vi "Template UIP Path.vi"() -> (3 "Template UIP Path":path)   [LabVIEW 2020, in "UIM.lvlib" / "UIM.lvclass"]
uses:
  UIM.lvclass
  TemplateUIP/TemplateUIP.lvclass
  UIM.lvclass/UIM.ctl
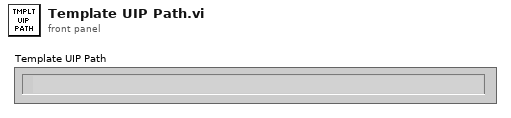
[diagram p1: front panel]
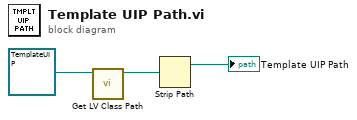
[diagram p0: block diagram]
diagram:
  n1 = call <vilib>:"Get LV Class Path.vi"("object"=refnum<class "TemplateUIP.lvclass"> refnum ("TemplateUIP.lvclass")) -> ("class path"=w2:path)  [unwired: 9 in, 1 out]
  n2 = Strip Path(path=w2) -> (stripped path=→"Template UIP Path":path)  [unwired: 1 out]
